vi "Pre Launch Init.vi"(11 "Cursor Digitizer in":refnum<class "Cursor Digitizer.lvclass">) -> (0 "error out":errorcluster, 3 "Cursor Digitizer out":refnum<class "Cursor Digitizer.lvclass">)   [LabVIEW 2016, in "Cursor Digitizer.lvclass"]
doc: "(<B>Filename</B>: Actor Framework.lvlib:Actor.lvclass:Pre Launch Init.vi)\n\nDefines behavior that occurs after the Launch Nested Actor method is invoked but before the actor's Actor Core method begins running.\n\nBy default, this method does nothing. A descendant class may override it to define behavior."
uses:
  Cursor Digitizer.lvclass
  Cursor Digitizer.lvclass/Cursor Digitizer.ctl
  <vilib>/ActorFramework/Actor/Actor.lvclass
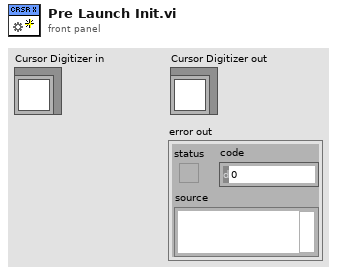
[diagram p1: front panel]
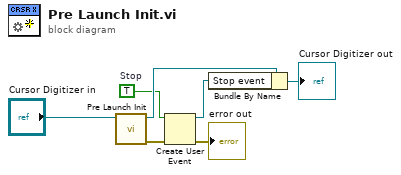
[diagram p0: block diagram]
diagram:
  w5 = TRUE  # Stop
  n1 = call-parent "Pre Launch Init.vi"("Actor in"="Cursor Digitizer in") -> ("error out"=w4:errorcluster, "Actor out"=w7:refnum<class "Cursor Digitizer.lvclass">)  [unwired: 9 in]
  n2 = Create User Event(user event datatype=w5, error in=w4) -> (user event=w1:refnum<user-event>, error out=→"error out":errorcluster)
  n3 = Bundle By Name(cluster=w7, "Stop event"=w1) -> (→"Cursor Digitizer out":refnum<class "Cursor Digitizer.lvclass">)
